vi "GV buffer label.vi"() -> ()   [LabVIEW 2017]
panel:
  in  "Memory":refnum<k21>
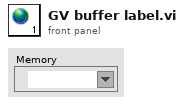
[diagram p1: front panel]
diagram:
